vi "RUSHArmControl.vi"(1 "In Cluster":T3) -> (0 "Out Cluster":T2)   [LabVIEW 2012]
uses:
  <vilib>/Rock Robotics/WPI/Relay/WPI_RelayValue.ctl
panel:
  in  "Max Speed":dbl=0.4
  in  "Setpoint P Gain":dbl=2.5
  in  "Manual P Gain":dbl=1.5
  in  "Vision P Gain":dbl=0.75
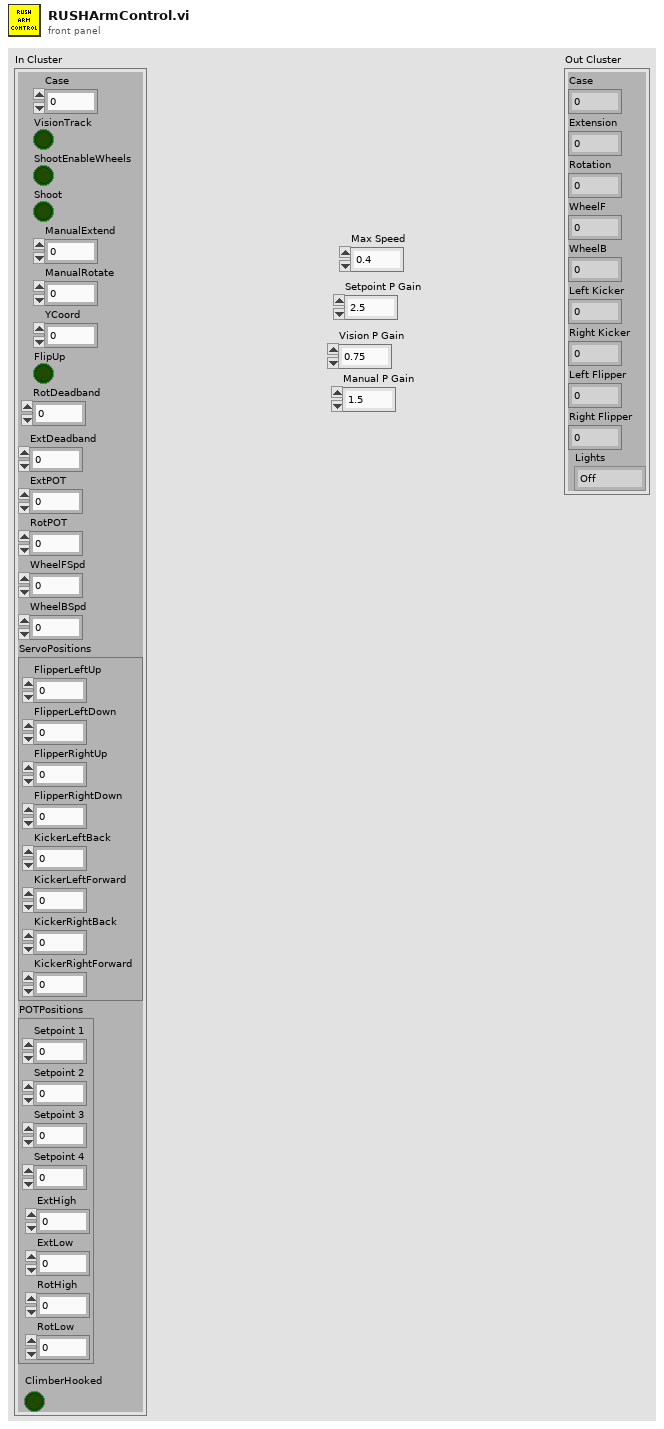
[diagram p1: front panel]
types:
  T1 = typedef "WPI_RelayValue.ctl" = enum16{"Off", "On", "Forward", "Reverse"}
  T2 = cluster{"Case":dbl, "Extension":dbl, "Rotation":dbl, "WheelF":dbl, "WheelB":dbl, "Left Kicker":dbl, "Right Kicker":dbl, "Left Flipper":dbl, "Right Flipper":dbl, "Lights":T1}
  T3 = cluster{"Case":dbl, "VisionTrack":bool, "ShootEnableWheels":bool, "Shoot":bool, "ManualExtend":dbl, "ManualRotate":dbl, "YCoord":dbl, "FlipUp":bool, "RotDeadband":dbl, "ExtDeadband":dbl, "ExtPOT":dbl, "RotPOT":dbl, "WheelFSpd":dbl, "WheelBSpd":dbl, "ServoPositions":cluster{"FlipperLeftUp":dbl, "FlipperLeftDown":dbl, "FlipperRightUp":dbl, "FlipperRightDown":dbl, "KickerLeftBack":dbl, "KickerLeftForward":dbl, "KickerRightBack":dbl, "KickerRightForward":dbl}, "POTPositions":cluster{"Setpoint 1":dbl, "Setpoint 2":dbl, "Setpoint 3":dbl, "Setpoint 4":dbl, "RotLow":dbl, "RotHigh":dbl, "ExtLow":dbl, "ExtHigh":dbl}, "ClimberHooked":bool}
  T4 = cluster{"FlipperLeftUp":dbl, "FlipperLeftDown":dbl, "FlipperRightUp":dbl, "FlipperRightDown":dbl, "KickerLeftBack":dbl, "KickerLeftForward":dbl, "KickerRightBack":dbl, "KickerRightForward":dbl}
  T5 = cluster{"Setpoint 1":dbl, "Setpoint 2":dbl, "Setpoint 3":dbl, "Setpoint 4":dbl, "RotLow":dbl, "RotHigh":dbl, "ExtLow":dbl, "ExtHigh":dbl}
  T6 = cluster{"t":dbl, "y":dbl, "y":dbl, "f":dbl, "f":dbl, "KickerLeftBack":dbl, "KickerRightBack":dbl, "FlipperLeftDown":dbl, "FlipperRightDown":dbl, "RelayValue":T1}
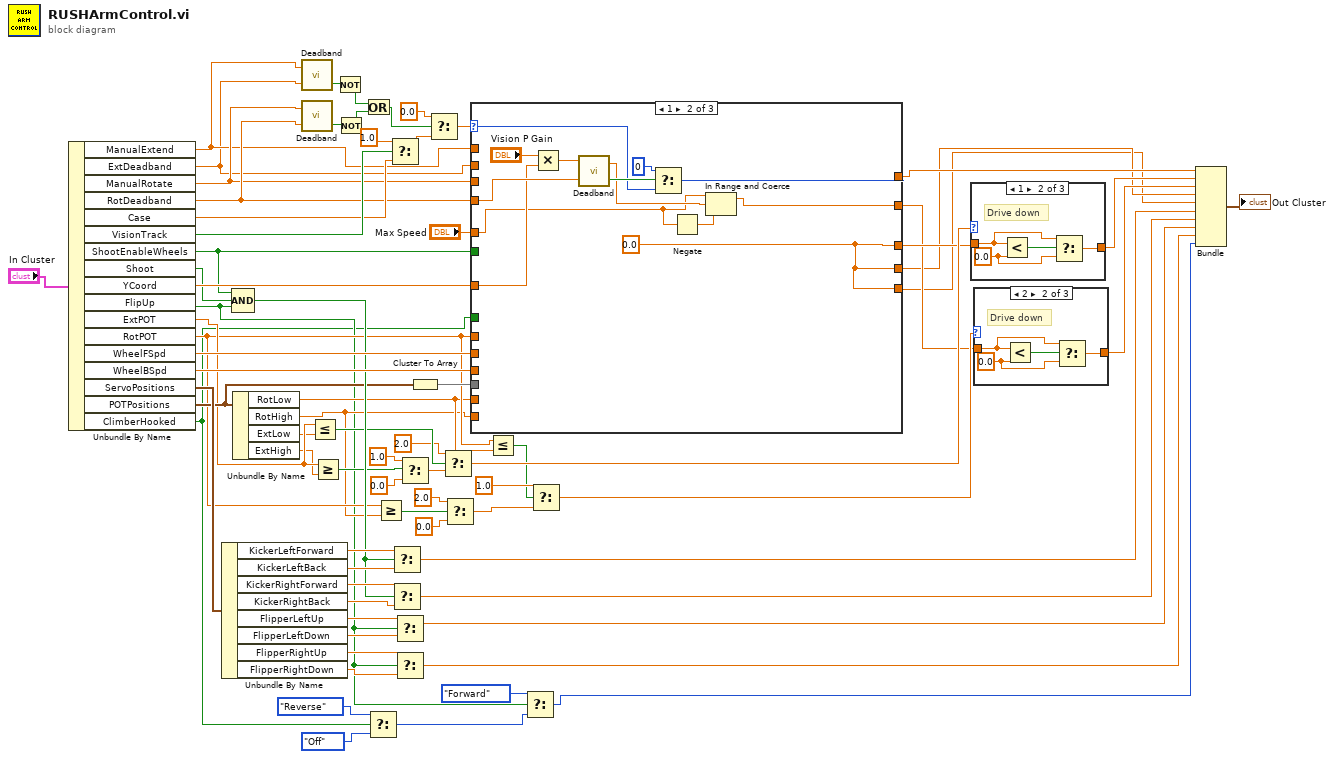
[diagram p0: block diagram]
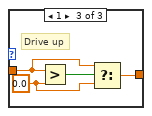
[diagram p3: hidden frame]
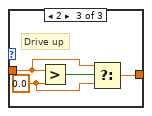
[diagram p5: hidden frame]
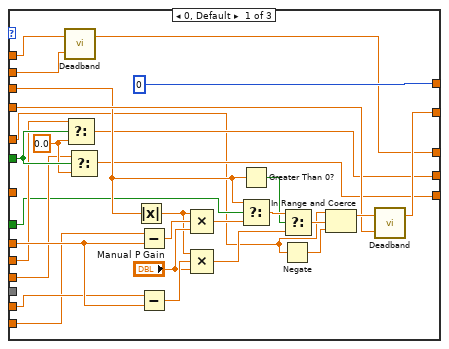
[diagram p6: hidden frame]
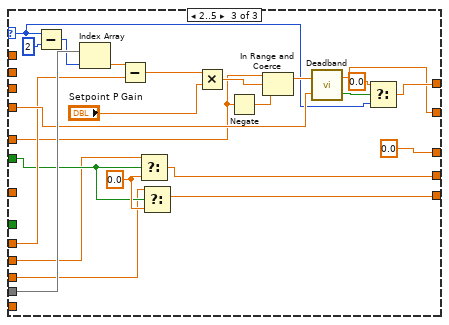
[diagram p7: hidden frame]
diagram:
  n1 = Unbundle By Name("In Cluster") -> ("ManualExtend"=w58:dbl, "ExtDeadband"=w57:dbl, "ManualRotate"=w59:dbl, "RotDeadband"=w61:dbl, "Case"=w62:dbl, "VisionTrack"=w63:bool, "ShootEnableWheels"=w52:bool, "Shoot"=w53:bool, "YCoord"=w60:dbl, "FlipUp"=w8:bool, "ExtPOT"=w35:dbl, "RotPOT"=w23:dbl, "WheelFSpd"=w56:dbl, "WheelBSpd"=w55:dbl, "ServoPositions"=w54:T4, "POTPositions"=w42:T5, "ClimberHooked"=w4:bool)
  n2 = Unbundle By Name(w54) -> ("KickerLeftForward"=w51:dbl, "KickerLeftBack"=w50:dbl, "KickerRightForward"=w49:dbl, "KickerRightBack"=w48:dbl, "FlipperLeftUp"=w46:dbl, "FlipperLeftDown"=w44:dbl, "FlipperRightUp"=w45:dbl, "FlipperRightDown"=w43:dbl)
  n3 = Compound Arithmetic op=AND(w52, w53, w8) -> (w47:bool)
  n4 = Unbundle By Name(w42) -> ("RotLow"=w22:dbl, "RotHigh"=w21:dbl, "ExtLow"=w34:dbl, "ExtHigh"=w33:dbl)
  n5 = call "Deadband.vi"("Deadband"=w57, "Input"=w58) -> ("In Deadband"=w68:bool)  [unwired: 1 out]
  n6 = call "Deadband.vi"("Deadband"=w61, "Input"=w59) -> ("In Deadband"=w67:bool)  [unwired: 1 out]
  n7 = Less Or Equal?(x=w35, y=w34) -> (x <= y?=w36:bool)
  n8 = Greater Or Equal?(x=w35, y=w33) -> (x >= y?=w40:bool)
  n9 = Not(x=w68) -> (.not. x?=w65:bool)
  n10 = Not(x=w67) -> (.not. x?=w66:bool)
  n11 = Or(x=w65, y=w66) -> (x .or. y?=w64:bool)
  n12 = Select(t=WPI_RelayValue."Reverse" ("RelayValue"), s=w4, f=WPI_RelayValue."Off" ("RelayValue")) -> (s? t:f=w1:T1)
  n13 = Greater Or Equal?(x=w23, y=w21) -> (x >= y?=w24:bool)
  n14 = Select(t=1.0, s=w63, f=w62) -> (s? t:f=w70:dbl)
  n15 = Select(t=w51, s=w47, f=w50) -> (s? t:f=w13:dbl)
  n16 = Select(t=w49, s=w47, f=w48) -> (s? t:f=w12:dbl)
  n17 = Select(t=w46, s=w8, f=w44) -> (s? t:f=w11:dbl)
  n18 = Select(t=w45, s=w8, f=w43) -> (s? t:f=w10:dbl)
  n19 = Select(t=1.0, s=w40, f=0.0) -> (s? t:f=w37:dbl)
  n20 = Cluster To Array(cluster=w42) -> (array=w41:dbl[])
  n21 = Select(t=0.0, s=w64, f=w70) -> (s? t:f=w73:dbl)
  n22 = Select(t=2.0, s=w36, f=w37) -> (s? t:f=w31:dbl)
  n23 = Select(t=2.0, s=w24, f=0.0) -> (s? t:f=w27:dbl)
  n24 = case shown="1" w73 {
    selector: w73 -> [_ w110 w126]
    tunnel: w61 -> [w88 w113 w130]
    tunnel: w60 -> [_ w112 _]
    tunnel: [0 ("t") w108 w125] -> w18
    tunnel: [w86 w103 w124] -> w19
    tunnel: w23 -> [w91 _ w129]
    tunnel: w22 -> [w90 _ _]
    tunnel: w21 -> [w89 _ _]
    tunnel: w59 -> [w87 _ _]
    tunnel: w58 -> [w84 _ _]
    tunnel: w57 -> [w83 _ _]
    tunnel: [w82 w107 0.0 ("Output")] -> w30
    tunnel: w52 -> [w81 _ w121]
    tunnel: w56 -> [w79 _ w119]
    tunnel: w55 -> [w78 _ w120]
    tunnel: [w77 w107 w118] -> w15
    tunnel: [w76 w107 w116] -> w14
    tunnel: w41 -> [_ _ w138]
    tunnel: w4 -> [w75 _ _]
    tunnel: "Max Speed" -> [w74 w104 w123]
    frame 0, Default {
      w80 = 0.0 ("f")
      n25 = call "Deadband.vi"("Deadband"=w83, "Input"=w84) -> ("Output"=w82:dbl)  [unwired: 1 out]
      n26 = Select(t=w79, s=w81, f=w80) -> (s? t:f=w77:dbl)
      n27 = Select(t=w78, s=w81, f=w80) -> (s? t:f=w76:dbl)
      n28 = Absolute Value(x=w87) -> (abs(x)=w96:dbl)
      n29 = Subtract(x=w89, y=w91) -> (x-y=w102:dbl)
      n30 = Subtract(x=w90, y=w91) -> (x-y=w101:dbl)
      n31 = Compound Arithmetic op=MULTIPLY(w96, w102, "Manual P Gain") -> (w99:dbl)
      n32 = Compound Arithmetic op=MULTIPLY(w96, w101, "Manual P Gain") -> (w97:dbl)
      n33 = Greater Than 0?(x=w87) -> (x > 0?=w95:bool)
      n34 = Select(t=w87, s=w75, f=w99) -> (s? t:f=w98:dbl)
      n35 = Negate(x=w74) -> (-x=w93:dbl)
      n36 = Select(t=w98, s=w95, f=w97) -> (s? t:f=w94:dbl)
      n37 = In Range and Coerce(upper limit=w74, x=w94, lower limit=w93) -> (coerced(x)=w92:dbl)  [unwired: 1 out]
      n38 = call "Deadband.vi"("Deadband"=w88, "Input"=w92) -> ("Output"=w86:dbl)  [unwired: 1 out]
    }
    frame 1 {
      w107 = 0.0 ("Output")
      n39 = Multiply(x="Vision P Gain", y=w112) -> (x*y=w114:dbl)
      n40 = call "Deadband.vi"("Deadband"=w113, "Input"=w114) -> ("In Deadband"=w111:bool, "Output"=w105:dbl)
      n41 = Select(t=0, s=w111, f=w110) -> (s? t:f=w108:i32)
      n42 = Negate(x=w104) -> (-x=w106:dbl)
      n43 = In Range and Coerce(upper limit=w104, x=w105, lower limit=w106) -> (coerced(x)=w103:dbl)  [unwired: 1 out]
    }
    frame 2..5 {
      w122 = 0.0 ("f")
      n44 = Subtract(x=w126, y=2) -> (x-y=w137:i32)
      n45 = Index Array(array=w138, index=w137) -> (element=w136:dbl)
      n46 = Subtract(x=w136, y=w129) -> (x-y=w135:dbl)
      n47 = Select(t=w119, s=w121, f=w122) -> (s? t:f=w118:dbl)
      n48 = Select(t=w120, s=w121, f=w122) -> (s? t:f=w116:dbl)
      n49 = Multiply(x=w135, y="Setpoint P Gain") -> (x*y=w132:dbl)
      n50 = Negate(x=w123) -> (-x=w133:dbl)
      n51 = In Range and Coerce(upper limit=w123, x=w132, lower limit=w133) -> (coerced(x)=w131:dbl)  [unwired: 1 out]
      n52 = call "Deadband.vi"("Deadband"=w130, "Input"=w131) -> ("In Deadband"=w128:bool, "Output"=w124:dbl)
      n53 = Select(t=0.0, s=w128, f=w126) -> (s? t:f=w125:dbl)
    }
  }
  n54 = Less Or Equal?(x=w23, y=w22) -> (x <= y?=w28:bool)
  n55 = Select(t=WPI_RelayValue."Forward" ("RelayValue"), s=w8, f=w1) -> (s? t:f=w6:T1)
  n56 = Select(t=1.0, s=w28, f=w27) -> (s? t:f=w20:dbl)
  n57 = case shown="1" w31 {
    tunnel: w30 -> [w140 w142 w146]
    tunnel: [w140 w141 w145] -> w17
    frame 0, Default {
      # "All good"
    }
    frame 1 {
      w143 = 0.0 ("y")
      # "Drive down"
      n58 = Less?(x=w142, y=w143) -> (x < y?=w144:bool)
      n59 = Select(t=w142, s=w144, f=w143) -> (s? t:f=w141:dbl)
    }
    frame 2 {
      w147 = 0.0 ("y")
      # "Drive up"
      n60 = Greater?(x=w146, y=w147) -> (0:w148:bool)
      n61 = Select(t=w146, s=w148, f=w147) -> (s? t:f=w145:dbl)
    }
  }
  n62 = case shown="2" w20 {
    tunnel: w19 -> [w149 w151 w155]
    tunnel: [w149 w150 w154] -> w16
    frame 0, Default {
      # "All good"
    }
    frame 2 {
      w152 = 0.0 ("y")
      # "Drive down"
      n63 = Less?(x=w151, y=w152) -> (x < y?=w153:bool)
      n64 = Select(t=w151, s=w153, f=w152) -> (s? t:f=w150:dbl)
    }
    frame 1 {
      w156 = 0.0 ("y")
      # "Drive up"
      n65 = Greater?(x=w155, y=w156) -> (0:w157:bool)
      n66 = Select(t=w155, s=w157, f=w156) -> (s? t:f=w154:dbl)
    }
  }
  n67 = Bundle("t"=w18, "y"=w17, "y"=w16, "f"=w15, "f"=w14, "KickerLeftBack"=w13, "KickerRightBack"=w12, "FlipperLeftDown"=w11, "FlipperRightDown"=w10, "RelayValue"=w6) -> (→"Out Cluster":T6)  [unwired: 1 in]
